vi "Dismiss All Errors.vi"(8 "error in (no error)":errorcluster, 11 "Error Manager in":refnum<class "Error Manager.lvclass">) -> (0 "error out":errorcluster, 3 "Error Manager out":refnum<class "Error Manager.lvclass">)   [LabVIEW 2026, in "TALOS.lvlib" / "Error Manager.lvlib" / "Error Manager.lvclass"]
uses:
  Error Manager.lvclass
  C:/LabVIEW Code/TALOS/talos/Father of all uServices/Father of all uServices/Father of all uServices.lvclass
  Error Info.ctl
  Father of all uServices/Father of all uServices/Father of all uServices.lvclass/Father of all uServices.ctl
  Ancestor/Ancestor/Ancestor.lvclass/Ancestor.ctl
  Error Manager.lvclass/Error Manager.ctl
  Common GUI v3/Common GUI v3/Error Listbox Msg.ctl
  Common GUI v3/Common GUI v3/Error Listbox Msg Action.ctl
  Guardian/Guardian/Requests.ctl
  Guardian/Guardian Messages/Requests from uServices Msg/Requests from uServices Msg.lvclass/Requests from uServices Msg.ctl
  Read Distributed flag.vi
  Write Array of Errors .vi
  Write Error indices mapping.vi
  Guardian/Guardian Messages/Requests from uServices Msg/Send Requests from uServices.vi
  Support VIs/Generate Error.vi
  FGV/Error Memory/Get Error Description.vi
  Support VIs/Get PC name.vi
  Ancestor/Ancestor/Read ID.vi
  Support VIs/Get Class Name.vi
  <vilib>/Utility/error.llb/Clear Errors.vi
  FGV/Error Memory/Error Memory Core.vi
  <vilib>/AdvancedString/Delimited String to 1D String Array.vi
  <vilib>/AdvancedString/Delimited String to 1D String Array (string).vi
  Support VIs/Circus Root Path.vi
  FGV/Error Memory/Error Crt Lvl checker.vi
  FGV/Error Memory/Error Memory Core.vi/40c8088d-b597-4017-91af-faa98e00292e.vi
  FGV/Error Memory/Error Memory Core.vi/d4a3ab98-063c-4e44-b43d-fbdcfe6c2be2.vi
  Father of all uServices/Father of all uServices/Father of all uServices.lvclass
  C:/LabVIEW Code/TALOS/builds/Actor Framework PPL/Actor Framework.lvlibp/1abvi3w/vi.lib/ActorFramework/Actor/Actor.lvclass
  Support VIs/Global Memory.vi
  <vilib>/Utility/LVClass/Get LV Class Name.vi
  Support VIs/Is in Packed Library.vi
  Support VIs/TALOS Root path.vi
  Support VIs/Read CSV worksheet.vi
  Support VIs/Global Constants.vi
  <vilib>/Utility/error.llb/General Error Handler.vi
  Support VIs/Error Log.vi
  builds/Actor Framework PPL/Actor Framework.lvlibp/1abvi3w/vi.lib/ActorFramework/Actor/Read Caller Enqueuer.vi
  builds/Actor Framework PPL/Actor Framework.lvlibp/1abvi3w/vi.lib/ActorFramework/Message Enqueuer/Enqueue.vi
  Ancestor/Ancestor/Ancestor.lvclass
  <vilib>/Comparison/Equal/Equal Functor/Equal Functor.lvclass
  Guardian/Guardian Messages/Requests from uServices Msg/Requests from uServices Msg.lvclass
  Common GUI v3/Common GUI v3/Common GUI v3.lvclass
  Guardian/Guardian/Guardian.lvclass
  TALOS.lvlib
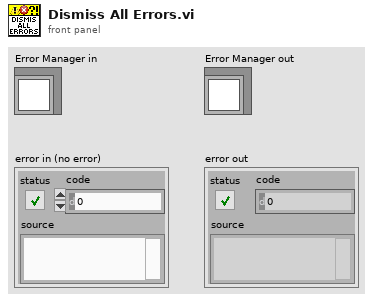
[diagram p1: front panel]
types:
  T1 = typedef "TALOS.lvlib/Guardian.lvlib/Guardian.lvclass/Requests.ctl" = enum16{"Ready to Launch", "Start RUN", "Stop RUN", "Update DAQ Params", "Update Error Listbox", "Update Run Status", "Update Kasli Log", "Run Stopped with Errors", "Switch uS View", "Dismiss All Errors"}
  T2 = typedef "TALOS.lvlib/Common GUI v3.lvlib/Common GUI v3.lvclass/Error Listbox Msg Action.ctl" = enum16{"Add", "Remove", "Clear"}
  T3 = typedef "TALOS.lvlib/Common GUI v3.lvlib/Common GUI v3.lvclass/Error Listbox Msg.ctl" = cluster{"Action":T2, "Error Info":T4}
  T4 = typedef "TALOS.lvlib/Error Manager.lvlib/Error Manager.lvclass/Error Info.ctl" = cluster{"error out":errorcluster, "Time Stamp":timestamp, "Machine Name":string, "GUID":string}
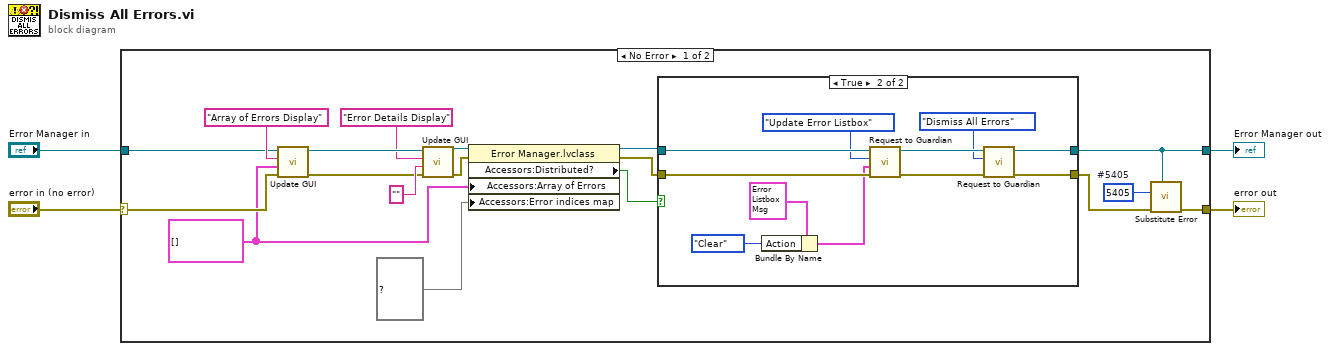
[diagram p0: block diagram]
diagram:
  n1 = case shown="No Error" "error in (no error)" {
    selector: "error in (no error)" -> [w15 w36]
    tunnel: [w18 w37] -> w4
    tunnel: [w17 w36] -> w3
    tunnel: "Error Manager in" -> [w5 w37]
    frame No Error {
      w7 = T4[] [] ("error constant")
      w16 = 5405  # #5405
      n2 = call "Update GUI.vi"("error in (no error)"=w15, "Data"=w7, "GUI Item Name"="Array of Errors Display" ("FP Item Name"), "uService Template in"=w5) -> ("error out"=w21:errorcluster, "uService Template out"=w20:refnum<class "Error Manager.lvclass">)  [unwired: 6 in]
      n3 = call "Update GUI.vi"("error in (no error)"=w21, "Data"="", "GUI Item Name"="Error Details Display", "uService Template in"=w20) -> ("error out"=w11:errorcluster, "uService Template out"=w12:refnum<class "Error Manager.lvclass">)  [unwired: 6 in]
      n4 = property class="Error Manager.lvclass"(reference=w12, error in=w11, "Accessors:Array of Errors "=w7, "Accessors:Error indices map"=map{i32, i32} {} ("Error indices mapping")) -> (reference out=w10:refnum<class "Error Manager.lvclass">, error out=w9:errorcluster, "Accessors:Distributed?"=w8:bool)
      n5 = case shown="True" w8 {
        tunnel: w9 -> [w23 w35]
        tunnel: w10 -> [w24 w34]
        tunnel: [w24 w28] -> w18
        tunnel: [w23 w26] -> w13
        frame False {
        }
        frame True {
          n6 = Bundle By Name(cluster=T3 {"Action"=enum."Add", "Error Info"={"error out"={"status"=FALSE, "code"=0, "source"=""}, "Time Stamp"=timestamp(0 s since 1904-01-01), "Machine Name"="", "GUID"=""}} ("Error Listbox Msg"), "Action"=Error_Listbox_Msg_Action."Clear") -> (w31:T3)
          n7 = call "Request to Guardian.vi"("error in (no error)"=w35, "Data"=w31, "Requests"=Requests."Update Error Listbox", "Father of all uServices in"=w34) -> ("error out"=w27:errorcluster, "Father of all uServices out"=w29:refnum<class "Error Manager.lvclass">)  [unwired: 6 in]
          n8 = call "Request to Guardian.vi"("error in (no error)"=w27, "Requests"=Requests."Dismiss All Errors", "Father of all uServices in"=w29) -> ("error out"=w26:errorcluster, "Father of all uServices out"=w28:refnum<class "Error Manager.lvclass">)  [unwired: 7 in]
        }
      }
      n9 = call "Substitute Error.vi"("LabVIEW Object"=w18, "error in (no error)"=w13, "Error Code"=w16) -> ("error out"=w17:errorcluster)  [unwired: 8 in]
    }
    frame Error {
    }
  }
  "Error Manager out" <- w4
  "error out" <- w3
